vi "Populate Attr Priv.vi"(6 "Item Indent":i32, 7 "Data Types Dict":variant, 8 "error in":errorcluster, 9 "Attribute Values":variant[](array[variant]), 10 "Attribute Names":string[](array[string]), 11 "Unique ID":string) -> (0 "error out":errorcluster, 1 "Attr Items":T1(array[cluster]))   [LabVIEW 2020, in "NI_VIAnCFGDataStructure.lvlib" / "Tree.lvclass"]
uses:
  <vilib>/addons/analyzer/VIAnCFGDataStructure/Tree Manager/Tree.lvclass
  <vilib>/addons/analyzer/VIAnCFGDataStructure/Tree Data/Tree Data.lvclass
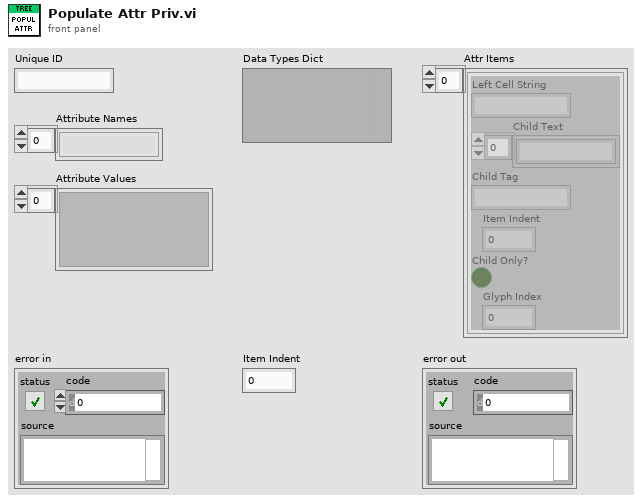
[diagram p1: front panel]
types:
  T1 = cluster{"Left Cell String":string, "Child Text":string[], "Child Tag":string, "Item Indent":i32, "Child Only?":bool, "Glyph Index":i32}[]
  T2 = cluster{"Left Cell String":string, "Child Text":string[], "Child Tag":string, "Item Indent":i32, "Child Only?":bool, "Glyph Index":i32}
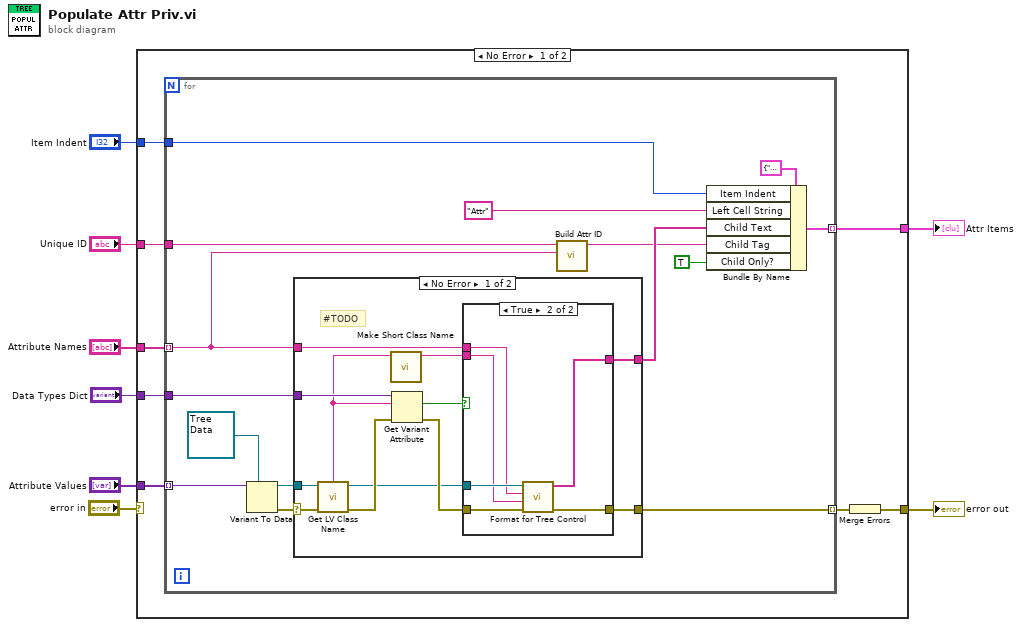
[diagram p0: block diagram]
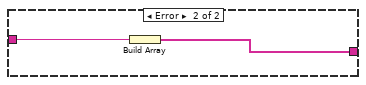
[diagram p3: hidden frame]
diagram:
  n1 = case shown="No Error" "error in" {
    selector: "error in" -> [_ w52]
    tunnel: "Unique ID" -> [w16 _]
    tunnel: "Attribute Names" -> [w15 _]
    tunnel: "Attribute Values" -> [w14 _]
    tunnel: "Data Types Dict" -> [w13 _]
    tunnel: [w11 w52] -> w4
    tunnel: "Item Indent" -> [w10 _]
    tunnel: [w9 _] -> w1
    frame No Error {
      n2 = for {
        tunnel: w15 -> [w28] mode=indexing
        tunnel: w16 -> [w19]
        tunnel: w14 -> [w31] mode=indexing
        tunnel: w13 -> [w27]
        tunnel: [w25] -> w12 mode=indexing
        tunnel: w10 -> [w18]
        tunnel: [w17] -> w9 mode=indexing
        n3 = Variant To Data(type=refnum<class "Tree Data.lvclass"> refnum ("Tree Data.lvclass"), Variant=w31) -> (data=w30:refnum<class "Tree Data.lvclass">, error out=w29:errorcluster)  [unwired: 1 in]
        n4 = case shown="No Error" w29 {
          selector: w29 -> [w42 _]
          tunnel: w30 -> [w37 _]
          tunnel: [w35 w50] -> w21
          tunnel: w28 -> [w36 w51]
          tunnel: w27 -> [w41 _]
          tunnel: [w34 _] -> w25
          frame No Error {
            # "#TODO"
            n5 = call <vilib>:"Get LV Class Name.vi"("error in (no error)"=w42, "object"=w37) -> ("error out"=w40:errorcluster, "class name"=w32:string)  [unwired: 8 in]
            n6 = call <vilib>:"Make Short Class Name.vi"("Class Name"=w32) -> ("Shortened Class Name"=w33:string)  [unwired: 10 in]
            n7 = Get Variant Attribute(Variant=w41, name=w32, error in=w40) -> (found=w38:bool, error out=w39:errorcluster)  [unwired: 1 in, 2 out]
            n8 = case shown="True" w38 {
              tunnel: w39 -> [w43 w48]
              tunnel: w37 -> [_ w49]
              tunnel: w36 -> [_ w47]
              tunnel: w33 -> [_ w46]
              tunnel: [_ w44] -> w35
              tunnel: [w43 w45] -> w34
              frame False {
              }
              frame True {
                n9 = call-dynamic "Format for Tree Control.vi"("Error In"=w48, "Class Name"=w46, "Attr Name"=w47, "Tree Data"=w49) -> ("Error Out"=w45:errorcluster, "Child Text"=w44:string[])  [unwired: 6 in]
              }
            }
          }
          frame Error {
            n10 = Build Array(w51) -> (w50:string[])
          }
        }
        n11 = call <vilib>:"Build Attr ID.vi"("Attr Name"=w28, "Unique ID"=w19) -> ("Attr ID Out"=w20:string)  [unwired: 9 in]
        n12 = Bundle By Name(cluster=T2 {"Left Cell String"="", "Child Text"=[], "Child Tag"="", "Item Indent"=0, "Child Only?"=FALSE, "Glyph Index"=0} ("Item"), "Item Indent"=w18, "Left Cell String"="Attr", "Child Text"=w21, "Child Tag"=w20, "Child Only?"=TRUE) -> (w17:T2)
      }
      n13 = Merge Errors(w12) -> (w11:errorcluster)
    }
    frame Error {
    }
  }
  "error out" <- w4
  "Attr Items" <- w1
